vi "Parse Description.vi"(0 "Description":string, 5 "XML Values to Parse":string[](array[string]), 11 "error in (no error) 2":errorcluster) -> (4 "Descritption without XML":string, 6 "XML Values":string[](array[string]), 8 "String Bounds of Matches":T1(array[cluster]), 15 "error out":errorcluster)   [LabVIEW 2017, in "CL_G3_VIComponentBuilder.lvlib"]
doc: "Parses out rhw xml tags specified in \"XML Values to Parse\" from a body of text. Returns the body without the xml that was specified. Returns the XML values specified."
uses:
  CL_G3_VIComponentBuilder.lvlib
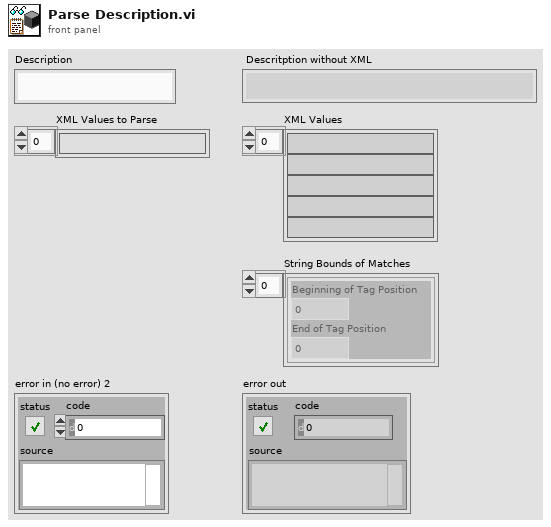
[diagram p1: front panel]
types:
  T1 = cluster{"Beginning of Tag Position":i32, "End of Tag Position":i32}[]
  T2 = cluster{"Beginning of Tag Position":i32, "End of Tag Position":i32}
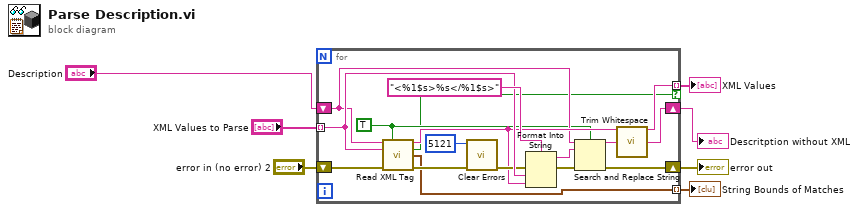
[diagram p0: block diagram]
diagram:
  n1 = for {
    shift-right: [w11] -> w4
    shift-left: "Description" -> [w16]
    tunnel: "XML Values to Parse" -> [w22] mode=indexing
    shift-right: [w13] -> w5
    shift-left: "error in (no error) 2" -> [w18]
    tunnel: [w17] -> w2 mode=indexing if=w8
    tunnel: [w9] -> w1 mode=indexing
    w10 = TRUE ("ignore case? (F)")
    n2 = call "Read XML Tag.vi"("XML String"=w16, "ignore case? (F)"=w10, "Tag"=w22, "error in (no error)"=w18) -> ("XML Tag Contents"=w17:string, "Found"=w8:bool, "String Bounds of Match"=w9:T2, "error out"=w20:errorcluster)  [unwired: 8 in]
    n3 = call <vilib>:"Clear Errors.vi"("error in (no error)"=w20, "specific error code to clear (0: all)"=5121) -> ("error out"=w19:errorcluster)  [unwired: 4 in, 1 out]
    n4 = Format Into String(format string="<%1$s>%s</%1$s>", error in=w19, w22, w17) -> (resulting string=w15:string, error out=w14:errorcluster)  [unwired: 1 in]
    n5 = Search and Replace String(case sensitive?=w10, input string=w16, search string=w15, error in=w14) -> (result string=w12:string, error out=w13:errorcluster)  [unwired: 4 in, 2 out]
    n6 = call <vilib>:"Trim Whitespace.vi"("string"=w12) -> ("trimmed string"=w11:string)  [unwired: 1 in]
  }
  "Descritption without XML" <- w4
  "error out" <- w5
  "XML Values" <- w2
  "String Bounds of Matches" <- w1
